vi "ShooterMotor.vi"(7 "RelayDevRef":T1, 8 "InnerRollerMtrRef":T5={"DeviceStatus"={"status"=FALSE, "code"=0, "source"=""}, "Type"=enum."PWM", "PWM"={"PWM Channel"=enum."PWM 4", "DeadBand"={"Name"="Victor", "maxPositivePwm"=1527, "minPositivePwm"=1014, "centerPwm"=1007, "maxNegativePwm"=1000, "minNegativePwm"=526, "angularRange"=0}}, "CAN"={"Device Number"=0, "Control Mode"=enum."Percent VBus", "Semaphore"=refnum, "Max Vout"=0.0, "TalonSRX Control Mode"=enum."Percent VBus"}, "Invert"=FALSE}, 9 "OuterRollerMtrRef":T5={"DeviceStatus"={"status"=FALSE, "code"=0, "source"=""}, "Type"=enum."PWM", "PWM"={"PWM Channel"=enum."PWM 5", "DeadBand"={"Name"="Victor", "maxPositivePwm"=1527, "minPositivePwm"=1014, "centerPwm"=1007, "maxNegativePwm"=1000, "minNegativePwm"=526, "angularRange"=0}}, "CAN"={"Device Number"=0, "Control Mode"=enum."Percent VBus", "Semaphore"=refnum, "Max Vout"=0.0, "TalonSRX Control Mode"=enum."Percent VBus"}, "Invert"=FALSE}, 10 "BottomShooterWheelMtrRef":T5={"DeviceStatus"={"status"=FALSE, "code"=0, "source"=""}, "Type"=enum."PWM", "PWM"={"PWM Channel"=enum."PWM 2", "DeadBand"={"Name"="Victor", "maxPositivePwm"=1527, "minPositivePwm"=1014, "centerPwm"=1007, "maxNegativePwm"=1000, "minNegativePwm"=526, "angularRange"=0}}, "CAN"={"Device Number"=0, "Control Mode"=enum."Percent VBus", "Semaphore"=refnum, "Max Vout"=0.0, "TalonSRX Control Mode"=enum."Percent VBus"}, "Invert"=FALSE}, 11 "UpperShooterWheelMtrRef":T5={"DeviceStatus"={"status"=FALSE, "code"=0, "source"=""}, "Type"=enum."PWM", "PWM"={"PWM Channel"=enum."PWM 3", "DeadBand"={"Name"="Victor", "maxPositivePwm"=1527, "minPositivePwm"=1014, "centerPwm"=1007, "maxNegativePwm"=1000, "minNegativePwm"=526, "angularRange"=0}}, "CAN"={"Device Number"=0, "Control Mode"=enum."Percent VBus", "Semaphore"=refnum, "Max Vout"=0.0, "TalonSRX Control Mode"=enum."Percent VBus"}, "Invert"=FALSE}) -> (0 "InnerRollerMtrRef":T5={"DeviceStatus"={"status"=FALSE, "code"=0, "source"=""}, "Type"=enum."PWM", "PWM"={"PWM Channel"=enum."PWM 4", "DeadBand"={"Name"="Victor", "maxPositivePwm"=1527, "minPositivePwm"=1014, "centerPwm"=1007, "maxNegativePwm"=1000, "minNegativePwm"=526, "angularRange"=0}}, "CAN"={"Device Number"=0, "Control Mode"=enum."Percent VBus", "Semaphore"=refnum, "Max Vout"=0.0, "TalonSRX Control Mode"=enum."Percent VBus"}, "Invert"=FALSE}, 1 "OuterRollerMtrRef":T5={"DeviceStatus"={"status"=FALSE, "code"=0, "source"=""}, "Type"=enum."PWM", "PWM"={"PWM Channel"=enum."PWM 5", "DeadBand"={"Name"="Victor", "maxPositivePwm"=1527, "minPositivePwm"=1014, "centerPwm"=1007, "maxNegativePwm"=1000, "minNegativePwm"=526, "angularRange"=0}}, "CAN"={"Device Number"=0, "Control Mode"=enum."Percent VBus", "Semaphore"=refnum, "Max Vout"=0.0, "TalonSRX Control Mode"=enum."Percent VBus"}, "Invert"=FALSE}, 2 "BottomShooterWheelMtrRef":T5={"DeviceStatus"={"status"=FALSE, "code"=0, "source"=""}, "Type"=enum."PWM", "PWM"={"PWM Channel"=enum."PWM 2", "DeadBand"={"Name"="Victor", "maxPositivePwm"=1527, "minPositivePwm"=1014, "centerPwm"=1007, "maxNegativePwm"=1000, "minNegativePwm"=526, "angularRange"=0}}, "CAN"={"Device Number"=0, "Control Mode"=enum."Percent VBus", "Semaphore"=refnum, "Max Vout"=0.0, "TalonSRX Control Mode"=enum."Percent VBus"}, "Invert"=FALSE}, 3 "UpperShootWheelMtrRef":T5={"DeviceStatus"={"status"=FALSE, "code"=0, "source"=""}, "Type"=enum."PWM", "PWM"={"PWM Channel"=enum."PWM 3", "DeadBand"={"Name"="Victor", "maxPositivePwm"=1527, "minPositivePwm"=1014, "centerPwm"=1007, "maxNegativePwm"=1000, "minNegativePwm"=526, "angularRange"=0}}, "CAN"={"Device Number"=0, "Control Mode"=enum."Percent VBus", "Semaphore"=refnum, "Max Vout"=0.0, "TalonSRX Control Mode"=enum."Percent VBus"}, "Invert"=FALSE}, 5 "RelayDevRef 2":T1)   [LabVIEW 2015]
uses:
  <vilib>/Rock Robotics/WPI/MotorControl/WPI_MotorControlDeviceRef.ctl
  <vilib>/Rock Robotics/WPI/MotorControl/WPI_MotorControlType.ctl
  <vilib>/Rock Robotics/SystemInterfaces/DIO/FPGA_DIOPWMChannel.ctl
  <vilib>/Rock Robotics/WPI/PWM/WPI_PWMDeadband.ctl
  <vilib>/Rock Robotics/WPI/CAN/Jaguar/SubVIs/WPI_CANJaguar_ControlMode.ctl
  <vilib>/Rock Robotics/WPI/CAN/TalonSRX/WPI_CANTalonSRX_APIControlMode.ctl
  <vilib>/Rock Robotics/WPI/Relay/WPI_RelayDevRef.ctl
  <vilib>/Rock Robotics/SystemInterfaces/DIO/FPGA_DIORelayChannel.ctl
  <vilib>/Rock Robotics/WPI/Relay/WPI_RelayDirection.ctl
  <vilib>/Rock Robotics/Network Tables/NT Read Number.vi
  Robot Values.vi
  <vilib>/Rock Robotics/Network Tables/NT Write Boolean.vi
  <vilib>/Rock Robotics/Network Tables/NT Read Boolean.vi
  <vilib>/addons/control/pid/pid.llb/PID (DBL).vi
  <vilib>/addons/control/pid/NI_PID_pid.lvlib
  <vilib>/ptbypt/NI_PtbyPt.lvlib
  <vilib>/Rock Robotics/WPI/Relay/WPI_RelayValue.ctl
panel:
  in  "Shooter Wait":dbl=0.75 format="%#_13g"
  in  "Shooter Power":dbl=0.65
  in  "Top Wheel Speed Multiplier":dbl=0.8
  in  "Beater Bar Reverse Speed":dbl=-0.33
  in  "Eject Speed":dbl=-0.85
  in  "Time Target (s)":dbl=1.0 format="%#_13g"
  in  "shooter wheel setpoint":dbl=55.0 format="%.2f"
  out "Elapsed Time (s)":dbl=4.24501895904541
  in  "Beater Bar Speed":dbl=0.75
  in  "shooter wheel speed tolerance":dbl=5.0
  in  "Shooter Wheel PID gains":T4={"proportional gain (Kc)"=0.024999999999999994, "integral time (Ti, min)"=0.0, "derivative time (Td, min)"=0.0} {"derivative time (Td, min)" format="%.3f"; "integral time (Ti, min)" format="%.3f"; "proportional gain (Kc)" format="%.3f"}
  # "May need adjusted"
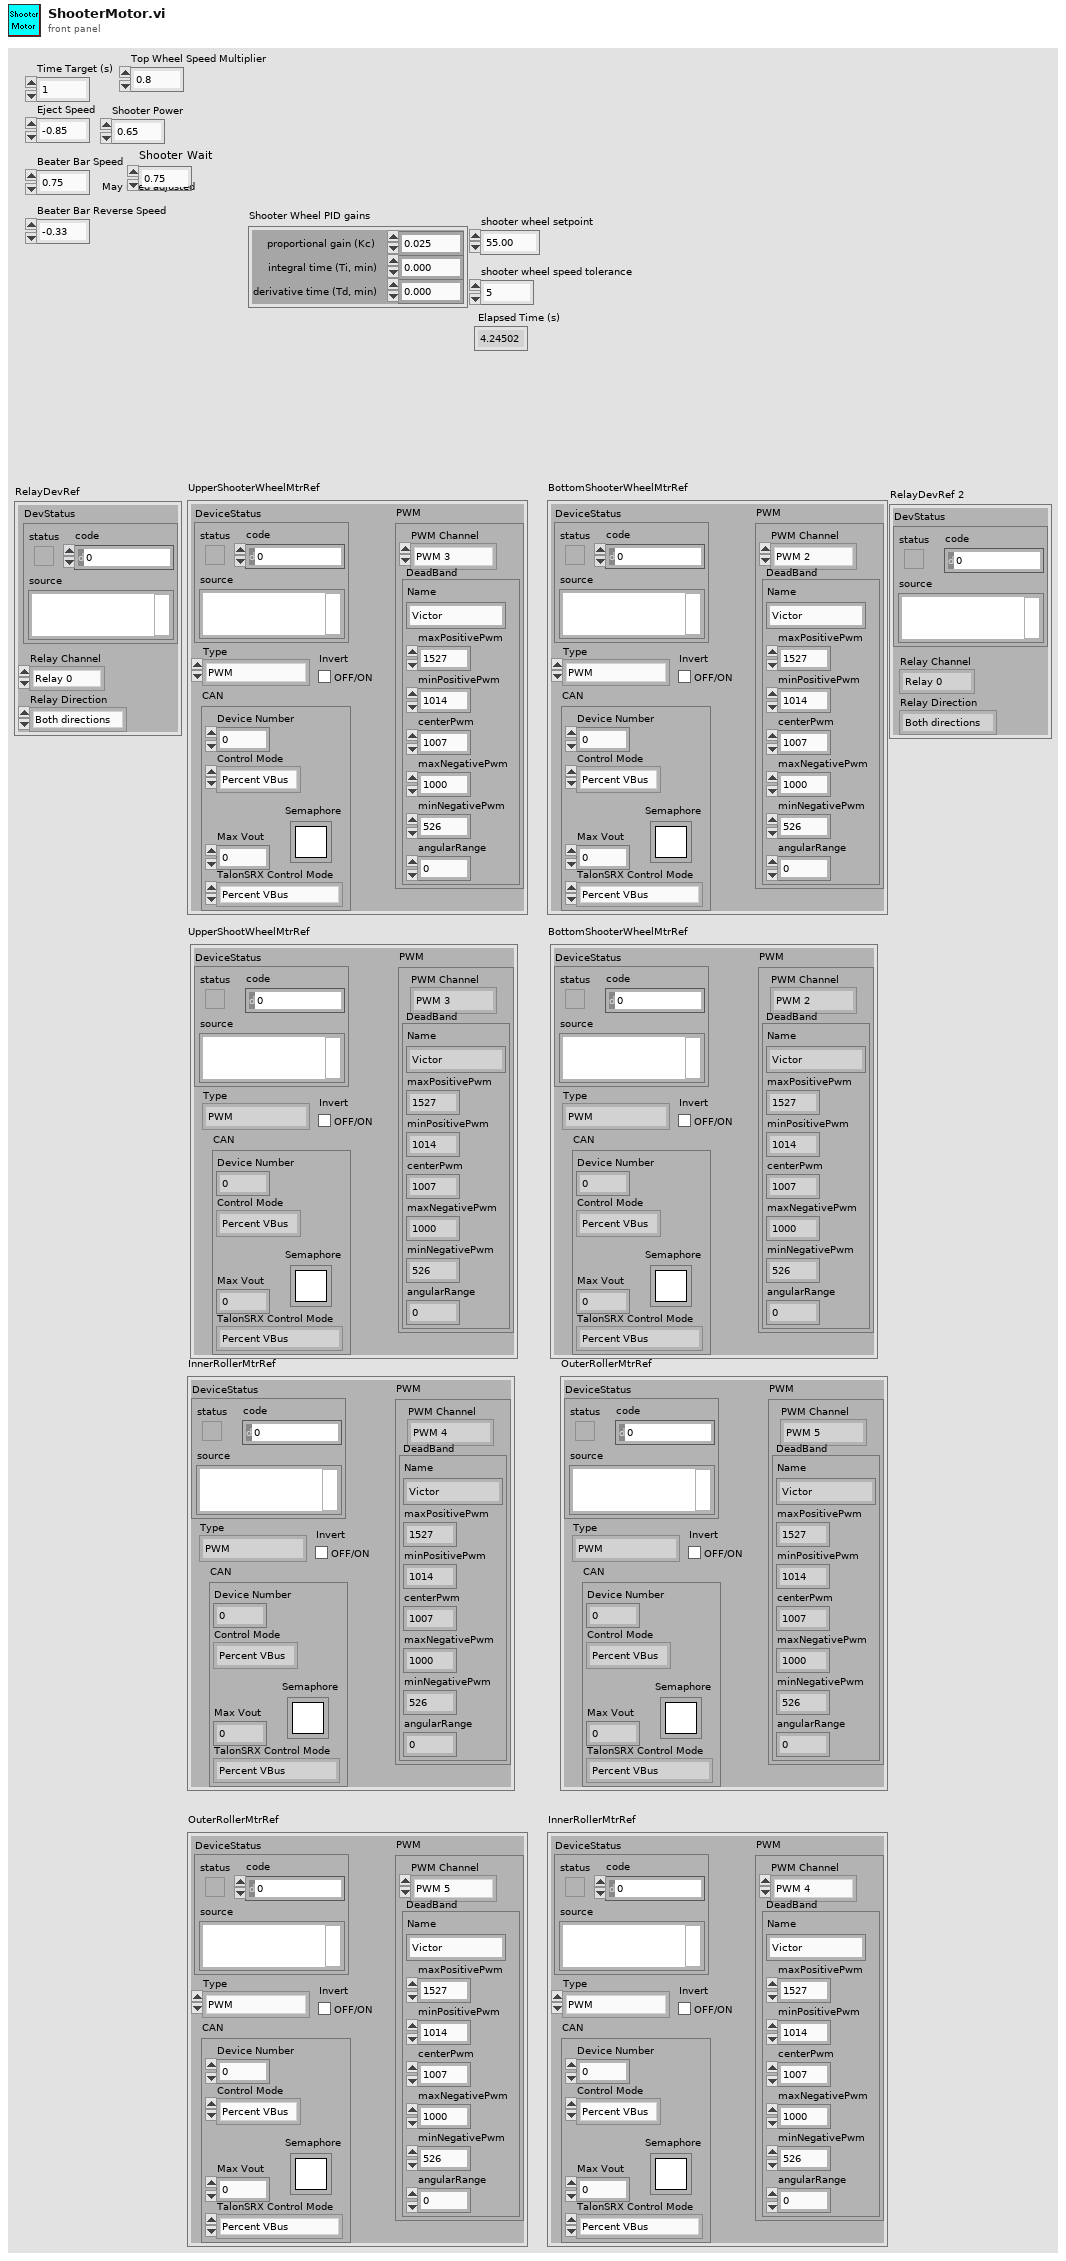
[diagram p1: front panel]
types:
  T1 = typedef "WPI_RelayDevRef.ctl" = cluster{"DevStatus":errorcluster, "Relay Channel":T2, "Relay Direction":T3}
  T2 = typedef "FPGA_DIORelayChannel.ctl" = enum8{"Relay 0", "Relay 1", "Relay 2", "Relay 3", "Invalid"}
  T3 = typedef "WPI_RelayDirection.ctl" = enum16{"Both directions", "Forward only", "Reverse only"}
  T4 = cluster{"proportional gain (Kc)":dbl, "integral time (Ti, min)":dbl, "derivative time (Td, min)":dbl}
  T5 = typedef "WPI_MotorControlDeviceRef.ctl" = cluster{"DeviceStatus":errorcluster, "Type":T6, "PWM":cluster{"PWM Channel":T7, "DeadBand":T8}, "CAN":cluster{"Device Number":u8, "Control Mode":T9, "Semaphore":T10, "Max Vout":dbl, "TalonSRX Control Mode":T11}, "Invert":bool}
  T6 = typedef "WPI_MotorControlType.ctl" = enum16{"PWM", "CAN", "CANTalonSRX"}
  T7 = typedef "FPGA_DIOPWMChannel.ctl" = enum8{"PWM 0", "PWM 1", "PWM 2", "PWM 3", "PWM 4", "PWM 5", "PWM 6", "PWM 7", "PWM 8", "PWM 9", "PWM MXP 0", "PWM MXP 1", "PWM MXP 2", "PWM MXP 3", "PWM MXP 4", "PWM MXP 5", "PWM MXP 6", "PWM MXP 7", "PWM MXP 8", "PWM MXP 9", "Invalid"}
  T8 = typedef "WPI_PWMDeadband.ctl" = cluster{"Name":string, "maxPositivePwm":i32, "minPositivePwm":i32, "centerPwm":i32, "maxNegativePwm":i32, "minNegativePwm":i32, "angularRange":u16}
  T9 = typedef "WPI_CANJaguar_ControlMode.ctl" = enum8{"Percent VBus", "Current", "Speed", "Position", "Voltage"}
  T10 = typedef "Semaphore RefNum" = refnum<k1>
  T11 = typedef "WPI_CANTalonSRX_APIControlMode.ctl" = enum8{"Percent VBus", "Speed", "Position", "Slave", "Unchanged / Invalid", "Voltage Compensation", "Current", "Motion Profile"}
  T12 = typedef "Robot Values.ctl" = cluster{"Drive Motors":cluster{"Left Motor Value":dbl, "Right Motor Value":dbl, "Left Motor Encoder":dbl, "Right Motor Encoder":dbl, "High/Low Gear":bool}, "Sensors":cluster{"Gyro Angle":dbl, "Photoeye":bool, "Ultrasonic Range":dbl, "Shooter Speed Encoder":dbl, "Accelerometer Value":dbl, "Flashlight":bool, "Target Distance":dbl, "Target X Value":dbl, "Reset Gyro?":bool}, "Arms":cluster{"Desired Arm Position":dbl, "Left Arm Encoder":dbl, "Right Arm Encoder":dbl, "Left Arm Lower Limit":bool, "Right Arm Lower Limit":bool, "Initialize Arm Position?":bool}, "Acquisition and Scoring":cluster{"Acquiring?":bool, "Current Speed":dbl, "Setpoint Speed":dbl, "Prep Wheels":bool, "Shoot":bool, "Low Eject":bool, "Reverse Shooter Wheel":bool}, "Hanging":cluster{"Pivot Arms":dbl, "PTO":bool, "Left Pivot Encoder":dbl, "Right Pivot Encoder":dbl, "Hanging Pin":bool}}
  T13 = typedef "WPI_RelayValue.ctl" = enum16{"Off", "On", "Forward", "Reverse"}
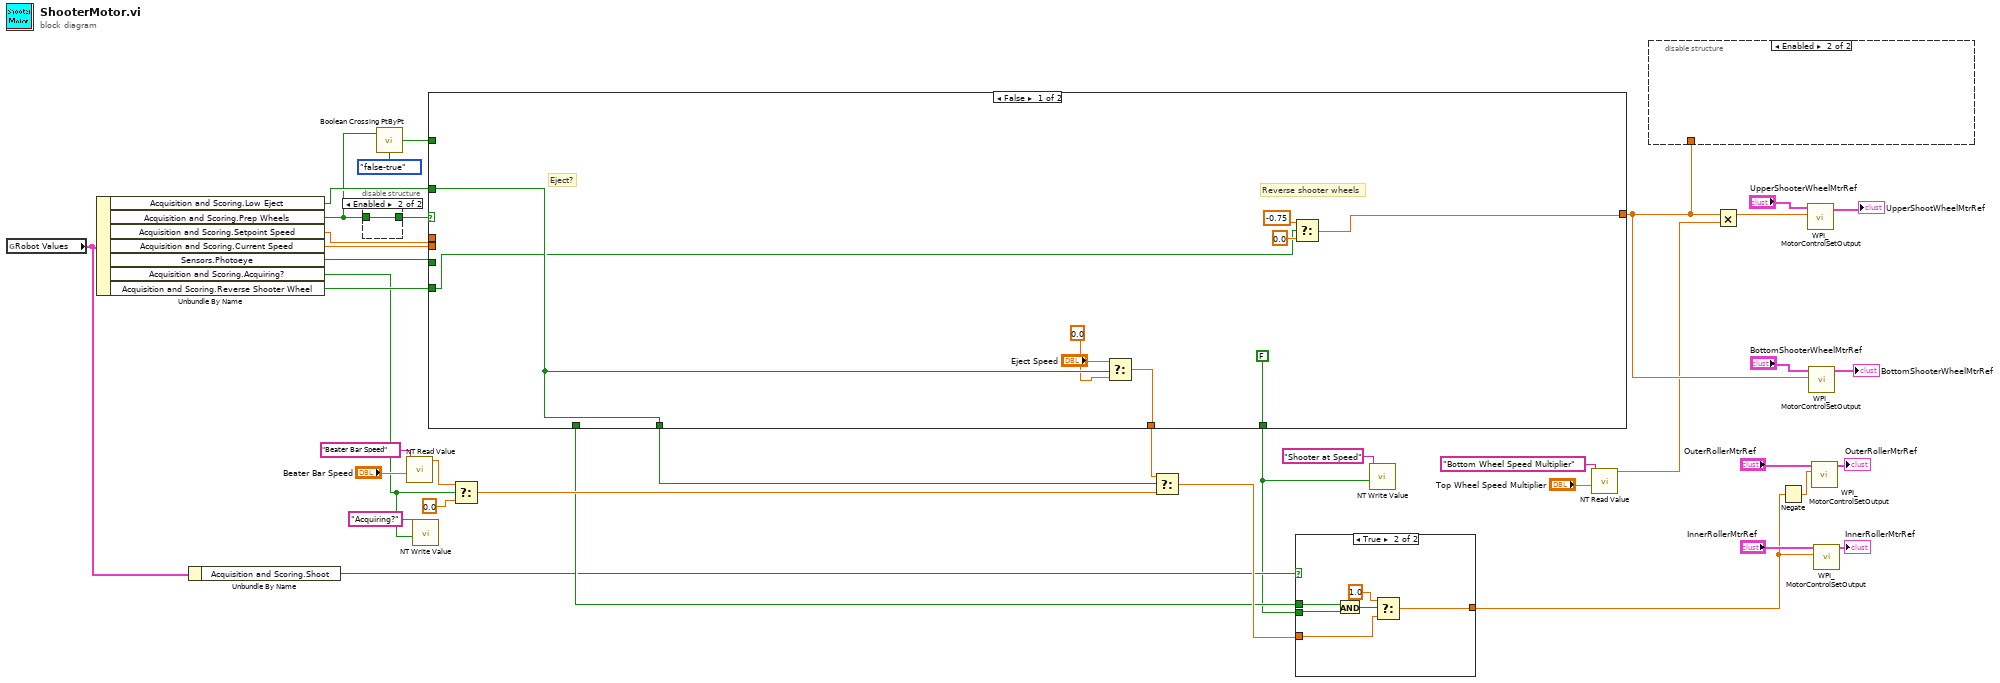
[diagram p0: block diagram]
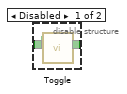
[diagram p2: hidden frame]
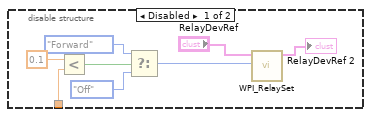
[diagram p3: hidden frame]
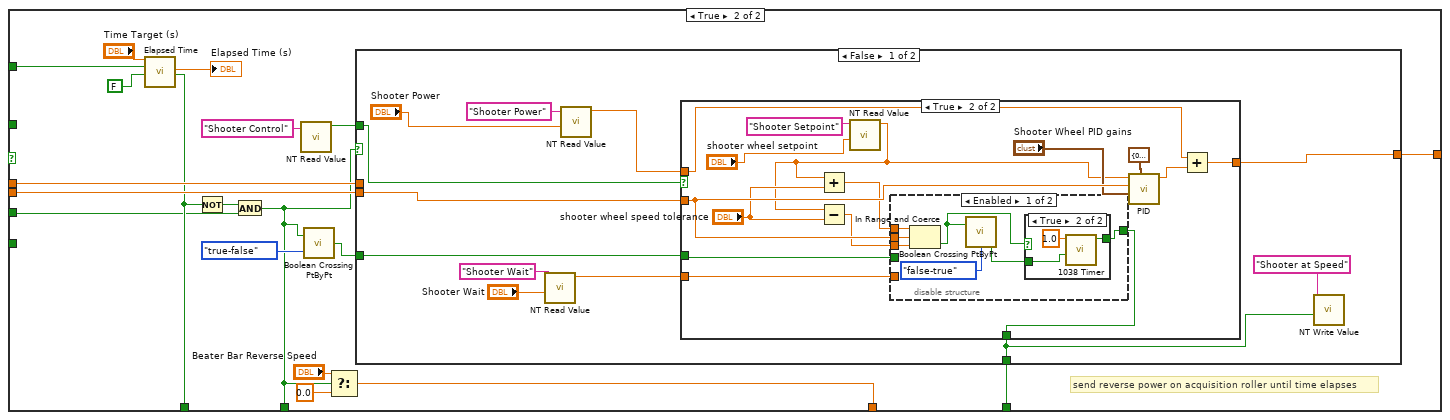
[diagram p5: hidden frame]
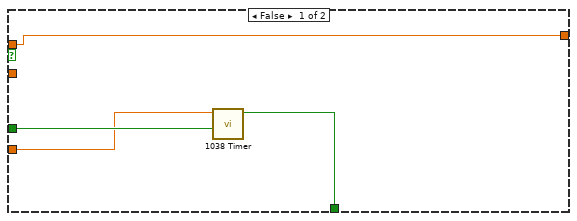
[diagram p6: hidden frame]
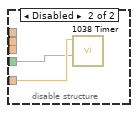
[diagram p8: hidden frame]
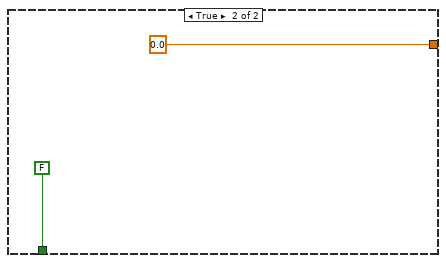
[diagram p9: hidden frame]
diagram:
  n1 = global read "Robot Values.vi" "Robot Values"() -> (w25:T12)
  n2 = Unbundle By Name(w25) -> ("Acquisition and Scoring.Low Eject"=w26:bool, "Acquisition and Scoring.Prep Wheels"=w7:bool, "Acquisition and Scoring.Setpoint Speed"=w39:dbl, "Acquisition and Scoring.Current Speed"=w30:dbl, "Sensors.Photoeye"=w29:bool, "Acquisition and Scoring.Acquiring?"=w10:bool, "Acquisition and Scoring.Reverse Shooter Wheel"=w17:bool)
  n3 = Unbundle By Name(w25) -> ("Acquisition and Scoring.Shoot"=w18:bool)
  n4 = disable-structure shown="Enabled" {
    disable-tunnel: w7 -> [w41 w42]
    disable-tunnel: [w40 w42] -> w16
    frame Disabled {
      n5 = call "Toggle.vi"("Input"=w41) -> ("output"=w40:bool)  [unwired: 10 in]
    }
    frame Enabled {
    }
  }
  n6 = call <vilib>:"Boolean Crossing PtByPt.vi"("direction"=enum16{"either", "false-true", "true-false"}."false-true", "input"=w7) -> ("crossing"=w6:bool)  [unwired: 1 in]
  n7 = call-poly <vilib>:"NT Read Value.vi"("Default Value"="Beater Bar Speed", "Name"="Beater Bar Speed") -> ("Numeric"=w13:dbl)  [unwired: 8 in, 1 out]
  n8 = call-poly <vilib>:"NT Write Value.vi"("Boolean"=w10, "Name"="Acquiring?") -> ()  [unwired: 9 in, 1 out]
  n9 = case shown="False" w16 {
    tunnel: w39 -> [_ w70]
    tunnel: w30 -> [_ w69]
    tunnel: [w45 w68] -> w5
    tunnel: [FALSE ("In Range?") w67] -> w1
    tunnel: w26 -> [w50 _]
    tunnel: [w50 w56] -> w24
    tunnel: w29 -> [_ w58]
    tunnel: [_ w62] -> w21
    tunnel: [w49 w61] -> w19
    tunnel: w17 -> [w43 _]
    tunnel: w6 -> [_ w52]
    frame False {
      # "Reverse shooter wheels"
      # "Eject?"
      n10 = Select(t="Eject Speed", s=w50, f=0.0) -> (s? t:f=w49:dbl)
      n11 = Select(t=-0.75, s=w43, f=0.0 ("output")) -> (s? t:f=w45:dbl)
    }
    frame True {
      # "send reverse power on acquisition roller until time elapses"
      n12 = call "Elapsed Time"("Time Target (s)"="Time Target (s)", "Reset"=w52, "Auto Reset"=FALSE) -> ("Elapsed Time (s)"=→"Elapsed Time (s)":dbl, "Time has Elapsed"=w62:bool)  [unwired: 9 in, 6 out]
      n13 = Not(x=w62) -> (.not. x?=w63:bool)
      n14 = And(x=w63, y=w58) -> (x .and. y?=w56:bool)
      n15 = call-poly <vilib>:"NT Read Value.vi"("Name"="Shooter Control") -> ("Boolean"=w54:bool)  [unwired: 9 in, 1 out]
      n16 = call <vilib>:"Boolean Crossing PtByPt.vi"("direction"=enum16{"either", "false-true", "true-false"}."true-false", "input"=w56) -> ("crossing"=w55:bool)  [unwired: 1 in]
      n17 = Select(t="Beater Bar Reverse Speed", s=w56, f=0.0) -> (s? t:f=w61:dbl)
      n18 = case shown="False" w56 {
        tunnel: w70 -> [_ _]
        tunnel: w69 -> [w81 _]
        tunnel: [w82 0.0 ("output")] -> w68
        tunnel: [w75 FALSE ("In Range?")] -> w67
        tunnel: w55 -> [w80 _]
        tunnel: w54 -> [w79 _]
        frame False {
          n19 = call-poly <vilib>:"NT Read Value.vi"("Default Value"="Shooter Wait", "Name"="Shooter Wait") -> ("Numeric"=w72:dbl)  [unwired: 8 in, 1 out]
          n20 = call-poly <vilib>:"NT Read Value.vi"("Default Value"="Shooter Power", "Name"="Shooter Power") -> ("Numeric"=w76:dbl)  [unwired: 8 in, 1 out]
          n21 = case shown="True" w79 {
            tunnel: [w84 w92] -> w82
            tunnel: w81 -> [_ w101]
            tunnel: w76 -> [w84 w90]
            tunnel: [w85 w87] -> w75
            tunnel: w80 -> [w86 w88]
            tunnel: w72 -> [w83 w89]
            frame False {
              n22 = call "1038 Timer.vi"("Reset?"=w86, "Time Target"=w83) -> ("Done?"=w85:bool)  [unwired: 9 in]
            }
            frame True {
              n23 = call-poly <vilib>:"NT Read Value.vi"("Default Value"="shooter wheel setpoint", "Name"="Shooter Setpoint") -> ("Numeric"=w94:dbl)  [unwired: 8 in, 1 out]
              n24 = Add(x=w94, y="shooter wheel speed tolerance") -> (x+y=w99:dbl)
              n25 = Subtract(x=w94, y="shooter wheel speed tolerance") -> (x-y=w98:dbl)
              n26 = disable-structure shown="Enabled" {
                disable-tunnel: w101 -> [w108 _]
                disable-tunnel: w99 -> [w107 _]
                disable-tunnel: w98 -> [w106 _]
                disable-tunnel: w89 -> [_ w113]
                disable-tunnel: w88 -> [_ w112]
                disable-tunnel: [w102 _] -> w87
                frame Enabled {
                  n27 = In Range and Coerce(upper limit=w107, x=w108, lower limit=w106) -> (In Range?=w104:bool)  [unwired: 1 out]
                  n28 = call <vilib>:"Boolean Crossing PtByPt.vi"("direction"=enum16{"either", "false-true", "true-false"}."false-true", "input"=w104) -> ("crossing"=w103:bool)  [unwired: 1 in]
                  n29 = case shown="True" w104 {
                    tunnel: [_ w110] -> w102
                    tunnel: w103 -> [_ w109]
                    frame False {
                    }
                    frame True {
                      n30 = call "1038 Timer.vi"("Reset?"=w109, "Time Target"=1.0) -> ("Done?"=w110:bool)  [unwired: 9 in]
                    }
                  }
                }
                frame Disabled {
                  n31 = call "1038 Timer.vi"("Reset?"=w112, "Time Target"=w113) -> ()  [unwired: 9 in, 1 out]
                }
              }
              n32 = call-poly <vilib>:"PID.vi"("output range"=cluster{"output high":dbl, "output low":dbl} {"output high"=0.1, "output low"=-0.1}, "PID gains"="Shooter Wheel PID gains", "process variable"=w101, "setpoint"=w94) -> ("output"=w91:dbl)  [unwired: 6 in, 1 out]
              n33 = Add(x=w90, y=w91) -> (x+y=w92:dbl)
            }
          }
          n34 = call-poly <vilib>:"NT Write Value.vi"("Boolean"=w75, "Name"="Shooter at Speed") -> ()  [unwired: 9 in, 1 out]
        }
        frame True {
        }
      }
    }
  }
  n35 = Select(t=w13, s=w10, f=0.0 ("t")) -> (s? t:f=w27:dbl)
  n36 = Select(t=w19, s=w24, f=w27) -> (s? t:f=w23:dbl)
  n37 = case shown="True" w18 {
    tunnel: [w116 w120] -> w22
    tunnel: w21 -> [_ w119]
    tunnel: w1 -> [_ w118]
    tunnel: w23 -> [w116 w117]
    frame False {
    }
    frame True {
      n38 = And(x=w119, y=w118) -> (x .and. y?=w122:bool)
      n39 = Select(t=1.0, s=w122, f=w117) -> (s? t:f=w120:dbl)
    }
  }
  n40 = call-poly <vilib>:"NT Write Value.vi"("Boolean"=w1, "Name"="Shooter at Speed") -> ()  [unwired: 9 in, 1 out]
  n41 = call-poly <vilib>:"NT Read Value.vi"("Default Value"="Top Wheel Speed Multiplier", "Name"="Bottom Wheel Speed Multiplier") -> ("Numeric"=w3:dbl)  [unwired: 8 in, 1 out]
  n42 = disable-structure shown="Enabled" {
    disable-tunnel: w5 -> [w130 _]
    frame Disabled {
      n43 = Less?(x=0.1 ("y"), y=w130) -> (x < y?=w128:bool)
      n44 = Select(t=WPI_RelayValue."Forward", s=w128, f=WPI_RelayValue."Off" ("RelayValue")) -> (s? t:f=w127:T13)
      n45 = call <vilib>:"WPI_RelaySet.vi"("RelayValue"=w127, "RelayDevRef"="RelayDevRef") -> ("RelayDevRef"=→"RelayDevRef 2":T1)  [unwired: 8 in, 1 out]
    }
    frame Enabled {
    }
  }
  n46 = Multiply(x=w5, y=w3) -> (x*y=w4:dbl)
  n47 = Negate(x=w22) -> (-x=w20:dbl)
  n48 = call <vilib>:"WPI_MotorControlSetOutput.vi"("Output"=w4, "MotorControlDevRef"="UpperShooterWheelMtrRef") -> ("MotorControlDevRef"=→"UpperShootWheelMtrRef":T5)  [unwired: 7 in, 2 out]
  n49 = call <vilib>:"WPI_MotorControlSetOutput.vi"("Output"=w5, "MotorControlDevRef"="BottomShooterWheelMtrRef") -> ("MotorControlDevRef"=→"BottomShooterWheelMtrRef":T5)  [unwired: 7 in, 2 out]
  n50 = call <vilib>:"WPI_MotorControlSetOutput.vi"("Output"=w20, "MotorControlDevRef"="OuterRollerMtrRef") -> ("MotorControlDevRef"=→"OuterRollerMtrRef":T5)  [unwired: 7 in, 2 out]
  n51 = call <vilib>:"WPI_MotorControlSetOutput.vi"("Output"=w22, "MotorControlDevRef"="InnerRollerMtrRef") -> ("MotorControlDevRef"=→"InnerRollerMtrRef":T5)  [unwired: 7 in, 2 out]
